vi "Weather Parse Test.vi"() -> ()   [LabVIEW 2020, in "CDM-Config.lvlib"] (continued)
        \"response\": \"Avoid\",\n                \"parameters\": {\n                    \"AWIPSidentifier\": [\n                        \"CWFWCZ\"\n                    ],\n                    \"WMOidentifier\": [\n                        \"FZAK52 PAFG 031247\"\n                    ],\n                    \"NWSheadline\": [\n                        \"GALE WARNING IN EFFECT THROUGH THIS MORNING... ...HEAVY FREEZING SPRAY WARNING IN EFFECT THROUGH LATE TONIGHT\"\n                    ],\n                    \"BLOCKCHANNEL\": [\n                        \"EAS\",\n                        \"NWEM\",\n                        \"CMAS\"\n                    ],\n                    \"VTEC\": [\n                        \"/O.NEW.PAFG.UP.W.8907.251203T1200Z-251204T1400Z/\"\n                    ],\n                    \"eventEndingTime\": [\n                        \"2025-12-04T05:00:00-09:00\"\n                    ]\n                },\n                \"scope\": \"Public\",\n                \"code\": \"IPAWSv1.0\",\n                \"language\": \"en-US\",\n                \"web\": \"http://www.weather.gov\",\n                \"eventCode\": {\n                    \"SAME\": [\n                        \"NWS\"\n                    ],\n                    \"NationalWeatherService\": [\n                        \"UPW\"\n                    ]\n                }\n            }\n        },\n        {\n            \"id\": \"https://api.weather.gov/alerts/urn:oid:2.49.0.1.840.0.c800d83de15e9a71d59e2d9241e36be98ce51c45.005.1\",\n            \"type\": \"Feature\",\n            \"geometry\": null,\n            \"properties\": {\n                \"@id\": \"https://api.weather.gov/alerts/urn:oid:2.49.0.1.840.0.c800d83de15e9a71d59e2d9241e36be98ce51c45.005.1\",\n                \"@type\": \"wx:Alert\",\n                \"id\": \"urn:oid:2.49.0.1.840.0.c800d83de15e9a71d59e2d9241e36be98ce51c45.005.1\",\n                \"areaDesc\": \"Flaxman Island to Demarcation Point out to 15 NM\",\n                \"geocode\": {\n                    \"SAME\": [\n                        \"058815\"\n                    ],\n                    \"UGC\": [\n                        \"PKZ815\"\n                    ]\n                },\n                \"affectedZones\": [\n                    \"https://api.weather.gov/zones/forecast/PKZ815\"\n                ],\n                \"references\": [],\n                \"sent\": \"2025-12-03T03:46:00-09:00\",\n                \"effective\": \"2025-12-03T03:45:00-09:00\",\n                \"onset\": \"2025-12-03T03:00:00-09:00\",\n                \"expires\": \"2025-12-03T18:00:00-09:00\",\n                \"ends\": \"2025-12-04T05:00:00-09:00\",\n                \"status\": \"Actual\",\n                \"messageType\": \"Alert\",\n                \"category\": \"Met\",\n                \"severity\": \"Minor\",\n                \"certainty\": \"Likely\",\n                \"urgency\": \"Expected\",\n                \"event\": \"Brisk Wind Advisory\",\n                \"sender\": \"w-nws.webmaster@noaa.gov\",\n                \"senderName\": \"NWS Fairbanks AK\",\n                \"headline\": \"Brisk Wind Advisory issued December 3 at 3:45AM AKST until December 4 at 5:00AM AKST by NWS Fairbanks AK\",\n                \"description\": \"Arctic Alaska Coastal Waters out 100 NM\\n\\nWind forecasts reflect the predominant speed and direction\\nexpected. Sea forecasts represent the average of the highest one-\\nthird of the combined wind-wave and swell height.\\n\\n.TODAY...W winds 25 kt.\\n.TONIGHT...W winds 25 kt.\\n.THU...W winds 10 kt.\\n.THU NIGHT...W winds 10 kt.\\n.FRI...NW winds 10 kt.\\n.FRI NIGHT...NW winds 10 kt.\\n.SAT...W winds 10 kt.\\n.SUN...W winds 10 kt.\",\n                \"instruction\": null,\n                \"response\": \"Avoid\",\n                \"parameters\": {\n                    \"AWIPSidentifier\": [\n                        \"CWFNSB\"\n                    ],\n                    \"WMOidentifier\": [\n                        \"FZAK51 PAFG 031246\"\n                    ],\n                    \"NWSheadline\": [\n                        \"BRISK WIND ADVISORY IN EFFECT THROUGH LATE TONIGHT\"\n                    ],\n                    \"BLOCKCHANNEL\": [\n                        \"EAS\",\n                        \"NWEM\",\n                        \"CMAS\"\n                    ],\n                    \"VTEC\": [\n                        \"/O.NEW.PAFG.BW.Y.7401.251203T1200Z-251204T1400Z/\"\n                    ],\n                    \"eventEndingTime\": [\n                        \"2025-12-04T05:00:00-09:00\"\n                    ]\n                },\n                \"scope\": \"Public\",\n                \"code\": \"IPAWSv1.0\",\n                \"language\": \"en-US\",\n                \"web\": \"http://www.weather.gov\",\n                \"eventCode\": {\n                    \"SAME\": [\n                        \"NWS\"\n                    ],\n                    \"NationalWeatherService\": [\n                        \"BWY\"\n                    ]\n                }\n            }\n        },\n        {\n            \"id\": \"https://api.weather.gov/alerts/urn:oid:2.49.0.1.840.0.c800d83de15e9a71d59e2d9241e36be98ce51c45.010.1\",\n            \"type\": \"Feature\",\n            \"geometry\": null,\n            \"properties\": {\n                \"@id\": \"https://api.weather.gov/alerts/urn:oid:2.49.0.1.840.0.c800d83de15e9a71d59e2d9241e36be98ce51c45.010.1\",\n                \"@type\": \"wx:Alert\",\n                \"id\": \"urn:oid:2.49.0.1.840.0.c800d83de15e9a71d59e2d9241e36be98ce51c45.010.1\",\n                \"areaDesc\": \"Flaxman Island to Demarcation Point from 15 to 75 NM\",\n                \"geocode\": {\n                    \"SAME\": [\n                        \"058861\"\n                    ],\n                    \"UGC\": [\n                        \"PKZ861\"\n                    ]\n                },\n                \"affectedZones\": [\n                    \"https://api.weather.gov/zones/forecast/PKZ861\"\n                ],\n                \"references\": [],\n                \"sent\": \"2025-12-03T03:46:00-09:00\",\n                \"effective\": \"2025-12-03T03:45:00-09:00\",\n                \"onset\": \"2025-12-03T03:00:00-09:00\",\n                \"expires\": \"2025-12-03T18:00:00-09:00\",\n                \"ends\": \"2025-12-04T05:00:00-09:00\",\n                \"status\": \"Actual\",\n                \"messageType\": \"Alert\",\n                \"category\": \"Met\",\n                \"severity\": \"Minor\",\n                \"certainty\": \"Likely\",\n                \"urgency\": \"Expected\",\n                \"event\": \"Brisk Wind Advisory\",\n                \"sender\": \"w-nws.webmaster@noaa.gov\",\n                \"senderName\": \"NWS Fairbanks AK\",\n                \"headline\": \"Brisk Wind Advisory issued December 3 at 3:45AM AKST until December 4 at 5:00AM AKST by NWS Fairbanks AK\",\n                \"description\": \"Arctic Alaska Coastal Waters out 100 NM\\n\\nWind forecasts reflect the predominant speed and direction\\nexpected. Sea forecasts represent the average of the highest one-\\nthird of the combined wind-wave and swell height.\\n\\n.TODAY...W winds 25 kt.\\n.TONIGHT...W winds 25 kt.\\n.THU...W winds 15 kt.\\n.THU NIGHT...W winds 10 kt.\\n.FRI...NW winds 10 kt.\\n.FRI NIGHT...N winds 10 kt.\\n.SAT...NW winds 10 kt.\\n.SUN...NW winds 10 kt.\",\n                \"instruction\": null,\n                \"response\": \"Avoid\",\n                \"parameters\": {\n                    \"AWIPSidentifier\": [\n                        \"CWFNSB\"\n                    ],\n                    \"WMOidentifier\": [\n                        \"FZAK51 PAFG 031246\"\n                    ],\n                    \"NWSheadline\": [\n                        \"BRISK WIND ADVISORY IN EFFECT THROUGH LATE TONIGHT\"\n                    ],\n                    \"BLOCKCHANNEL\": [\n                        \"EAS\",\n                        \"NWEM\",\n                        \"CMAS\"\n                    ],\n                    \"VTEC\": [\n                        \"/O.NEW.PAFG.BW.Y.7402.251203T1200Z-251204T1400Z/\"\n                    ],\n                    \"eventEndingTime\": [\n                        \"2025-12-04T05:00:00-09:00\"\n                    ]\n                },\n                \"scope\": \"Public\",\n                \"code\": \"IPAWSv1.0\",\n                \"language\": \"en-US\",\n                \"web\": \"http://www.weather.gov\",\n                \"eventCode\": {\n                    \"SAME\": [\n                        \"NWS\"\n                    ],\n                    \"NationalWeatherService\": [\n                        \"BWY\"\n                    ]\n                }\n            }\n        },\n        {\n            \"id\": \"https://api.weather.gov/alerts/urn:oid:2.49.0.1.840.0.01783fcbff0a57acfaa8774dbd3d755b2c9bae1b.005.1\",\n            \"type\": \"Feature\",\n            \"geometry\": null,\n            \"properties\": {\n                \"@id\": \"https://api.weather.gov/alerts/urn:oid:2.49.0.1.840.0.01783fcbff0a57acfaa8774dbd3d755b2c9bae1b.005.1\",\n                \"@type\": \"wx:Alert\",\n                \"id\": \"urn:oid:2.49.0.1.840.0.01783fcbff0a57acfaa8774dbd3d755b2c9bae1b.005.1\",\n                \"areaDesc\": \"Boulder And Jefferson Counties Below 6000 Feet/West Broomfield County; North Douglas County Below 6000 Feet/Denver/West Adams and Arapahoe Counties/East Broomfield County; Elbert/Central and East Douglas Counties Above 6000 Feet\",\n                \"geocode\": {\n                    \"SAME\": [\n                        \"008013\",\n                        \"008014\",\n                        \"008059\",\n                        \"008001\",\n                        \"008005\",\n                        \"008031\",\n                        \"008035\",\n                        \"008039\"\n                    ],\n                    \"UGC\": [\n                        \"COZ039\",\n                        \"COZ040\",\n                        \"COZ041\"\n                    ]\n                },\n                \"affectedZones\": [\n                    \"https://api.weather.gov/zones/forecast/COZ039\",\n                    \"https://api.weather.gov/zones/forecast/COZ040\",\n                    \"https://api.weather.gov/zones/forecast/COZ041\"\n                ],\n                \"references\": [\n                    {\n                        \"@id\": \"https://api.weather.gov/alerts/urn:oid:2.49.0.1.840.0.dc493d5144a5e7b208e25eb0a352a3a4cb8daa39.005.1\",\n                        \"identifier\": \"urn:oid:2.49.0.1.840.0.dc493d5144a5e7b208e25eb0a352a3a4cb8daa39.005.1\",\n                        \"sender\": \"w-nws.webmaster@noaa.gov\",\n                        \"sent\": \"2025-12-02T14:37:00-07:00\"\n                    },\n                    {\n                        \"@id\": \"https://api.weather.gov/alerts/urn:oid:2.49.0.1.840.0.9981ab0aab6442180ca93df6a3f6876711e70914.004.1\",\n                        \"identifier\": \"urn:oid:2.49.0.1.840.0.9981ab0aab6442180ca93df6a3f6876711e70914.004.1\",\n                        \"sender\": \"w-nws.webmaster@noaa.gov\",\n                        \"sent\": \"2025-12-02T22:13:00-07:00\"\n                    }\n                ],\n                \"sent\": \"2025-12-03T05:02:00-07:00\",\n                \"effective\": \"2025-12-03T05:02:00-07:00\",\n                \"onset\": \"2025-12-03T05:02:00-07:00\",\n                \"expires\": \"2025-12-03T13:15:00-07:00\",\n                \"ends\": \"2025-12-03T18:00:00-07:00\",\n                \"status\": \"Actual\",\n                \"messageType\": \"Update\",\n                \"category\": \"Met\",\n                \"severity\": \"Moderate\",\n                \"certainty\": \"Likely\",\n                \"urgency\": \"Expected\",\n                \"event\": \"Winter Weather Advisory\",\n                \"sender\": \"w-nws.webmaster@noaa.gov\",\n                \"senderName\": \"NWS Denver CO\",\n                \"headline\": \"Winter Weather Advisory issued December 3 at 5:02AM MST until December 3 at 6:00PM MST by NWS Denver CO\",\n                \"description\": \"* WHAT...Snow. Additional snow accumulations between 1 and 4 inches,\\nwith storm totals ranging from 3 to 6 inches. The heavier totals\\nwill be west of I-25. Locally heavier amounts close to 8 inches\\nwill be possible at the base of the foothills.\\n\\n* WHERE...Boulder and Denver metro areas, Castle Rock, and Palmer\\nDivide.\\n\\n* WHEN...Until 6 PM MST this evening.\\n\\n* IMPACTS...Plan on slippery road conditions and slow travel. The\\nhazardous conditions will impact the Wednesday morning commute,\\nwith potential for slick roads to persist into the evening commute\\nas well.\",\n                \"instruction\": \"Slow down and use caution while traveling. The latest road conditions\\nfor Colorado can be obtained by calling 5 1 1 or by going to\\nwww.cotrip.org.\",\n                \"response\": \"Execute\",\n                \"parameters\": {\n                    \"AWIPSidentifier\": [\n                        \"WSWBOU\"\n                    ],\n                    \"WMOidentifier\": [\n                        \"WWUS45 KBOU 031202\"\n                    ],\n                    \"NWSheadline\": [\n                        \"WINTER WEATHER ADVISORY REMAINS IN EFFECT UNTIL 6 PM MST THIS EVENING\"\n                    ],\n                    \"BLOCKCHANNEL\": [\n                        \"EAS\",\n                        \"NWEM\",\n                        \"CMAS\"\n                    ],\n                    \"VTEC\": [\n                        \"/O.CON.KBOU.WW.Y.0029.000000T0000Z-251204T0100Z/\"\n                    ],\n                    \"eventEndingTime\": [\n                        \"2025-12-03T18:00:00-07:00\"\n                    ],\n                    \"expiredReferences\": [\n                        \"w-nws.webmaster@noaa.gov,urn:oid:2.49.0.1.840.0.a94969ba77db5be5a7a7221a7b90d8c1f14402d8.002.1,2025-12-02T02:53:00-07:00 w-nws.webmaster@noaa.gov,urn:oid:2.49.0.1.840.0.e69a2f297fcb0f2a4247bcda904ffb3742464c99.001.1,2025-12-01T13:52:00-07:00\"\n                    ]\n                },\n                \"scope\": \"Public\",\n                \"code\": \"IPAWSv1.0\",\n                \"language\": \"en-US\",\n                \"web\": \"http://www.weather.gov\",\n                \"eventCode\": {\n                    \"SAME\": [\n                        \"NWS\"\n                    ],\n                    \"NationalWeatherService\": [\n                        \"WWY\"\n                    ]\n                }\n            }\n        },\n        {\n            \"id\": \"https://api.weather.gov/alerts/urn:oid:2.49.0.1.840.0.01783fcbff0a57acfaa8774dbd3d755b2c9bae1b.003.1\",\n            \"type\": \"Feature\",\n            \"geometry\": null,\n            \"properties\": {\n                \"@id\": \"https://api.weather.gov/alerts/urn:oid:2.49.0.1.840.0.01783fcbff0a57acfaa8774dbd3d755b2c9bae1b.003.1\",\n                \"@type\": \"wx:Alert\",\n                \"id\": \"urn:oid:2.49.0.1.840.0.01783fcbff0a57acfaa8774dbd3d755b2c9bae1b.003.1\",\n                \"areaDesc\": \"Central and Southeast Park County\",\n                \"geocode\": {\n                    \"SAME\": [\n                        \"008093\"\n                    ],\n                    \"UGC\": [\n                        \"COZ037\"\n                    ]\n                },\n                \"affectedZones\": [\n                    \"https://api.weather.gov/zones/forecast/COZ037\"\n                ],\n                \"references\": [\n                    {\n                        \"@id\": \"https://api.weather.gov/alerts/urn:oid:2.49.0.1.840.0.dc493d5144a5e7b208e25eb0a352a3a4cb8daa39.002.1\",\n                        \"identifier\": \"urn:oid:2.49.0.1.840.0.dc493d5144a5e7b208e25eb0a352a3a4cb8daa39.002.1\",\n                        \"sender\": \"w-nws.webmaster@noaa.gov\",\n                        \"sent\": \"2025-12-02T14:37:00-07:00\"\n                    },\n                    {\n                        \"@id\": \"https://api.weather.gov/alerts/urn:oid:2.49.0.1.840.0.9981ab0aab6442180ca93df6a3f6876711e70914.005.1\",\n                        \"identifier\": \"urn:oid:2.49.0.1.840.0.9981ab0aab6442180ca93df6a3f6876711e70914.005.1\",\n                        \"sender\": \"w-nws.webmaster@noaa.gov\",\n                        \"sent\": \"2025-12-02T22:13:00-07:00\"\n                    }\n                ],\n                \"sent\": \"2025-12-03T05:02:00-07:00\",\n                \"effective\": \"2025-12-03T05:02:00-07:00\",\n                \"onset\": \"2025-12-03T05:02:00-07:00\",\n                \"expires\": \"2025-12-03T13:15:00-07:00\",\n                \"ends\": \"2025-12-03T20:00:00-07:00\",\n                \"status\": \"Actual\",\n                \"messageType\": \"Update\",\n                \"category\": \"Met\",\n                \"severity\": \"Moderate\",\n                \"certainty\": \"Likely\",\n                \"urgency\": \"Expected\",\n                \"event\": \"Winter Weather Advisory\",\n                \"sender\": \"w-nws.webmaster@noaa.gov\",\n                \"senderName\": \"NWS Denver CO\",\n                \"headline\": \"Winter Weather Advisory issued December 3 at 5:02AM MST until December 3 at 8:00PM MST by NWS Denver CO\",\n                \"description\": \"* WHAT...Snow expected. Total snow accumulations between 3 and 8\\ninches.\\n\\n* WHERE...South Park.\\n\\n* WHEN...Until 8 PM MST this evening.\\n\\n* IMPACTS...Travel will be hazardous with slippery road conditions.\",\n                \"instruction\": \"Slow down and use caution while traveling. The latest road conditions\\nfor Colorado can be obtained by calling 5 1 1 or by going to\\nwww.cotrip.org.\",\n                \"response\": \"Execute\",\n                \"parameters\": {\n                    \"AWIPSidentifier\": [\n                        \"WSWBOU\"\n                    ],\n                    \"WMOidentifier\": [\n                        \"WWUS45 KBOU 031202\"\n                    ],\n                    \"NWSheadline\": [\n                        \"WINTER WEATHER ADVISORY REMAINS IN EFFECT UNTIL 8 PM MST THIS EVENING\"\n                    ],\n                    \"BLOCKCHANNEL\": [\n                        \"EAS\",\n                        \"NWEM\",\n                        \"CMAS\"\n                    ],\n                    \"VTEC\": [\n                        \"/O.CON.KBOU.WW.Y.0029.000000T0000Z-251204T0300Z/\"\n                    ],\n                    \"eventEndingTime\": [\n                        \"2025-12-03T20:00:00-07:00\"\n                    ]\n                },\n                \"scope\": \"Public\",\n                \"code\": \"IPAWSv1.0\",\n                \"language\": \"en-US\",\n                \"web\": \"http://www.weather.gov\",\n                \"eventCode\": {\n                    \"SAME\": [\n                        \"NWS\"\n                    ],\n                    \"NationalWeatherService\": [\n                        \"WWY\"\n                    ]\n                }\n            }\n        },\n        {\n            \"id\": \"https://api.weather.gov/alerts/urn:oid:2.49.0.1.840.0.01783fcbff0a57acfaa8774dbd3d755b2c9bae1b.002.1\",\n            \"type\": \"Feature\",\n            \"geometry\": null,\n            \"properties\": {\n                \"@id\": \"https://api.weather.gov/alerts/urn:oid:2.49.0.1.840.0.01783fcbff0a57acfaa8774dbd3d755b2c9bae1b.002.1\",\n                \"@type\": \"wx:Alert\",\n                \"id\": \"urn:oid:2.49.0.1.840.0.01783fcbff0a57acfaa8774dbd3d755b2c9bae1b.002.1\",\n                \"areaDesc\": \"Jefferson and West Douglas Counties Above  6000 Feet/Gilpin/Clear Creek/Northeast Park Counties Below 9000 Feet\",\n                \"geocode\": {\n                    \"SAME\": [\n                        \"008019\",\n                        \"008035\",\n                        \"008047\",\n                        \"008059\",\n                        \"008093\"\n                    ],\n                    \"UGC\": [\n                        \"COZ036\"\n                    ]\n                },\n                \"affectedZones\": [\n                    \"https://api.weather.gov/zones/forecast/COZ036\"\n                ],\n                \"references\": [\n                    {\n                        \"@id\": \"https://api.weather.gov/alerts/urn:oid:2.49.0.1.840.0.dc493d5144a5e7b208e25eb0a352a3a4cb8daa39.004.1\",\n                        \"identifier\": \"urn:oid:2.49.0.1.840.0.dc493d5144a5e7b208e25eb0a352a3a4cb8daa39.004.1\",\n                        \"sender\": \"w-nws.webmaster@noaa.gov\",\n                        \"sent\": \"2025-12-02T14:37:00-07:00\"\n                    },\n                    {\n                        \"@id\": \"https://api.weather.gov/alerts/urn:oid:2.49.0.1.840.0.9981ab0aab6442180ca93df6a3f6876711e70914.002.1\",\n                        \"identifier\": \"urn:oid:2.49.0.1.840.0.9981ab0aab6442180ca93df6a3f6876711e70914.002.1\",\n                        \"sender\": \"w-nws.webmaster@noaa.gov\",\n                        \"sent\": \"2025-12-02T22:13:00-07:00\"\n                    }\n                ],\n                \"sent\": \"2025-12-03T05:02:00-07:00\",\n                \"effective\": \"2025-12-03T05:02:00-07:00\",\n                \"onset\": \"2025-12-03T05:02:00-07:00\",\n                \"expires\": \"2025-12-03T13:15:00-07:00\",\n                \"ends\": \"2025-12-03T18:00:00-07:00\",\n                \"status\": \"Actual\",\n                \"messageType\": \"Update\",\n                \"category\": \"Met\",\n                \"severity\": \"Moderate\",\n                \"certainty\": \"Likely\",\n                \"urgency\": \"Expected\",\n                \"event\": \"Winter Weather Advisory\",\n                \"sender\": \"w-nws.webmaster@noaa.gov\",\n                \"senderName\": \"NWS Denver CO\",\n                \"headline\": \"Winter Weather Advisory issued December 3 at 5:02AM MST until December 3 at 6:00PM MST by NWS Denver CO\",\n                \"description\": \"* WHAT...Snow. Additional snow accumulations between 3 and 8 inches,\\nbringing storm totals into the 6 to 11 inch range.\\n\\n* WHERE...The Southern Front Range Foothills.\\n\\n* WHEN...Until 6 PM MST this evening.\\n\\n* IMPACTS...Travel could be difficult. The hazardous conditions will\\nimpact the Wednesday morning and afternoon commutes.\",\n                \"instruction\": \"Slow down and use caution while traveling. The latest road conditions\\nfor Colorado can be obtained by calling 5 1 1 or by going to\\nwww.cotrip.org.\",\n                \"response\": \"Execute\",\n                \"parameters\": {\n                    \"AWIPSidentifier\": [\n                        \"WSWBOU\"\n                    ],\n                    \"WMOidentifier\": [\n                        \"WWUS45 KBOU 031202\"\n                    ],\n                    \"NWSheadline\": [\n                        \"WINTER WEATHER ADVISORY REMAINS IN EFFECT UNTIL 6 PM MST THIS EVENING\"\n                    ],\n                    \"BLOCKCHANNEL\": [\n                        \"EAS\",\n                        \"NWEM\",\n                        \"CMAS\"\n                    ],\n                    \"VTEC\": [\n                        \"/O.CON.KBOU.WW.Y.0029.000000T0000Z-251204T0100Z/\"\n                    ],\n                    \"eventEndingTime\": [\n                        \"2025-12-03T18:00:00-07:00\"\n                    ],\n                    \"expiredReferences\": [\n                        \"w-nws.webmaster@noaa.gov,urn:oid:2.49.0.1.840.0.a94969ba77db5be5a7a7221a7b90d8c1f14402d8.001.1,2025-12-02T02:53:00-07:00 w-nws.webmaster@noaa.gov,urn:oid:2.49.0.1.840.0.e69a2f297fcb0f2a4247bcda904ffb3742464c99.001.1,2025-12-01T13:52:00-07:00\"\n                    ]\n                },\n                \"scope\": \"Public\",\n                \"code\": \"IPAWSv1.0\",\n                \"language\": \"en-US\",\n                \"web\": \"http://www.weather.gov\",\n                \"eventCode\": {\n                    \"SAME\": [\n                        \"NWS\"\n                    ],\n                    \"NationalWeatherService\": [\n                        \"WWY\"\n                    ]\n                }\n            }\n        },\n        {\n            \"id\": \"https://api.weather.gov/alerts/urn:oid:2.49.0.1.840.0.01783fcbff0a57acfaa8774dbd3d755b2c9bae1b.001.1\",\n            \"type\": \"Feature\",\n            \"geometry\": null,\n            \"properties\": {\n                \"@id\": \"https://api.weather.gov/alerts/urn:oid:2.49.0.1.840.0.01783fcbff0a57acfaa8774dbd3d755b2c9bae1b.001.1\",\n                \"@type\": \"wx:Alert\",\n                \"id\": \"urn:oid:2.49.0.1.840.0.01783fcbff0a57acfaa8774dbd3d755b2c9bae1b.001.1\",\n                \"areaDesc\": \"Larimer and Boulder Counties Between 6000 and 9000 Feet\",\n                \"geocode\": {\n                    \"SAME\": [\n                        \"008013\",\n                        \"008069\"\n                    ],\n                    \"UGC\": [\n                        \"COZ035\"\n                    ]\n                },\n                \"affectedZones\": [\n                    \"https://api.weather.gov/zones/forecast/COZ035\"\n                ],\n                \"references\": [\n                    {\n                        \"@id\": \"https://api.weather.gov/alerts/urn:oid:2.49.0.1.840.0.dc493d5144a5e7b208e25eb0a352a3a4cb8daa39.003.1\",\n                        \"identifier\": \"urn:oid:2.49.0.1.840.0.dc493d5144a5e7b208e25eb0a352a3a4cb8daa39.003.1\",\n                        \"sender\": \"w-nws.webmaster@noaa.gov\",\n                        \"sent\": \"2025-12-02T14:37:00-07:00\"\n                    },\n                    {\n                        \"@id\": \"https://api.weather.gov/alerts/urn:oid:2.49.0.1.840.0.9981ab0aab6442180ca93df6a3f6876711e70914.001.1\",\n                        \"identifier\": \"urn:oid:2.49.0.1.840.0.9981ab0aab6442180ca93df6a3f6876711e70914.001.1\",\n                        \"sender\": \"w-nws.webmaster@noaa.gov\",\n                        \"sent\": \"2025-12-02T22:13:00-07:00\"\n                    }\n                ],\n                \"sent\": \"2025-12-03T05:02:00-07:00\",\n                \"effective\": \"2025-12-03T05:02:00-07:00\",\n                \"onset\": \"2025-12-03T05:02:00-07:00\",\n                \"expires\": \"2025-12-03T13:15:00-07:00\",\n                \"ends\": \"2025-12-03T18:00:00-07:00\",\n                \"status\": \"Actual\",\n                \"messageType\": \"Update\",\n                \"category\": \"Met\",\n                \"severity\": \"Moderate\",\n                \"certainty\": \"Likely\",\n                \"urgency\": \"Expected\",\n                \"event\": \"Winter Weather Advisory\",\n                \"sender\": \"w-nws.webmaster@noaa.gov\",\n                \"senderName\": \"NWS Denver CO\",\n                \"headline\": \"Winter Weather Advisory issued December 3 at 5:02AM MST until December 3 at 6:00PM MST by NWS Denver CO\",\n                \"description\": \"* WHAT...Snow. Additional snow accumulations between 2 and 4 inches,\\nbringing storm totals to between 3 and 9 inches. The heaviest\\namounts will be in the Boulder County Foothills, with lighter\\namounts in northern Larimer County.\\n\\n* WHERE...The Northern Front Range Foothills.\\n\\n* WHEN...Until 6 PM MST this evening.\\n\\n* IMPACTS...Travel could be difficult. The hazardous conditions will\\nimpact the Wednesday morning commute.\",\n                \"instruction\": \"Slow down and use caution while traveling. The latest road conditions\\nfor Colorado can be obtained by calling 5 1 1 or by going to\\nwww.cotrip.org.\",\n                \"response\": \"Execute\",\n                \"parameters\": {\n                    \"AWIPSidentifier\": [\n                        \"WSWBOU\"\n                    ],\n                    \"WMOidentifier\": [\n                        \"WWUS45 KBOU 031202\"\n                    ],\n                    \"NWSheadline\": [\n                        \"WINTER WEATHER ADVISORY REMAINS IN EFFECT UNTIL 6 PM MST THIS EVENING\"\n                    ],\n                    \"BLOCKCHANNEL\": [\n                        \"EAS\",\n                        \"NWEM\",\n                        \"CMAS\"\n                    ],\n                    \"VTEC\": [\n                        \"/O.CON.KBOU.WW.Y.0029.000000T0000Z-251204T0100Z/\"\n                    ],\n                    \"eventEndingTime\": [\n                        \"2025-12-03T18:00:00-07:00\"\n                    ]\n                },\n                \"scope\": \"Public\",\n                \"code\": \"IPAWSv1.0\",\n                \"language\": \"en-US\",\n                \"web\": \"http://www.weather.gov\",\n                \"eventCode\": {\n                    \"SAME\": [\n                        \"NWS\"\n                    ],\n                    \"NationalWeatherService\": [\n                        \"WWY\"\n                    ]\n                }\n            }\n        },\n        {\n            \"id\": \"https://api.weather.gov/alerts/urn:oid:2.49.0.1.840.0.01783fcbff0a57acfaa8774dbd3d755b2c9bae1b.004.1\",\n            \"type\": \"Feature\",\n            \"geometry\": null,\n            \"properties\": {\n                \"@id\": \"https://api.weather.gov/alerts/urn:oid:2.49.0.1.840.0.01783fcbff0a57acfaa8774dbd3d755b2c9bae1b.004.1\",\n                \"@type\": \"wx:Alert\",\n                \"id\": \"urn:oid:2.49.0.1.840.0.01783fcbff0a57acfaa8774dbd3d755b2c9bae1b.004.1\",\n                \"areaDesc\": \"Larimer County Below 6000 Feet/Northwest Weld County\",\n                \"geocode\": {\n                    \"SAME\": [\n                        \"008069\",\n                        \"008123\"\n                    ],\n                    \"UGC\": [\n                        \"COZ038\"\n                    ]\n                },\n                \"affectedZones\": [\n                    \"https://api.weather.gov/zones/forecast/COZ038\"\n                ],\n                \"references\": [\n                    {\n                        \"@id\": \"https://api.weather.gov/alerts/urn:oid:2.49.0.1.840.0.dc493d5144a5e7b208e25eb0a352a3a4cb8daa39.001.1\",\n                        \"identifier\": \"urn:oid:2.49.0.1.840.0.dc493d5144a5e7b208e25eb0a352a3a4cb8daa39.001.1\",\n                        \"sender\": \"w-nws.webmaster@noaa.gov\",\n                        \"sent\": \"2025-12-02T14:37:00-07:00\"\n                    },\n                    {\n                        \"@id\": \"https://api.weather.gov/alerts/urn:oid:2.49.0.1.840.0.9981ab0aab6442180ca93df6a3f6876711e70914.003.1\",\n                        \"identifier\": \"urn:oid:2.49.0.1.840.0.9981ab0aab6442180ca93df6a3f6876711e70914.003.1\",\n                        \"sender\": \"w-nws.webmaster@noaa.gov\",\n                        \"sent\": \"2025-12-02T22:13:00-07:00\"\n                    }\n                ],\n                \"sent\": \"2025-12-03T05:02:00-07:00\",\n                \"effective\": \"2025-12-03T05:02:00-07:00\",\n                \"onset\": \"2025-12-03T05:02:00-07:00\",\n                \"expires\": \"2025-12-03T13:15:00-07:00\",\n                \"ends\": \"2025-12-03T14:00:00-07:00\",\n                \"status\": \"Actual\",\n                \"messageType\": \"Update\",\n                \"category\": \"Met\",\n                \"severity\": \"Moderate\",\n                \"certainty\": \"Likely\",\n                \"urgency\": \"Expected\",\n                \"event\": \"Winter Weather Advisory\",\n                \"sender\": \"w-nws.webmaster@noaa.gov\",\n                \"senderName\": \"NWS Denver CO\",\n                \"headline\": \"Winter Weather Advisory issued December 3 at 5:02AM MST until December 3 at 2:00PM MST by NWS Denver CO\",\n                \"description\": \"* WHAT...Snow. Additional snow accumulations less than two inches,\\nwith storm totals mostly between 2 and 5 inches.\\n\\n* WHERE...Fort Collins and Loveland.\\n\\n* WHEN...Until 2 PM MST this afternoon.\\n\\n* IMPACTS...Plan on slippery road conditions and slow travel. The\\nhazardous conditions will impact the Wednesday morning commute,\\nwith potential for slick roads to persist into the evening commute\\nas well.\",\n                \"instruction\": \"Slow down and use caution while traveling. The latest road conditions\\nfor Colorado can be obtained by calling 5 1 1 or by going to\\nwww.cotrip.org.\",\n                \"response\": \"Execute\",\n                \"parameters\": {\n                    \"AWIPSidentifier\": [\n                        \"WSWBOU\"\n                    ],\n                    \"WMOidentifier\": [\n                        \"WWUS45 KBOU 031202\"\n                    ],\n                    \"NWSheadline\": [\n                        \"WINTER WEATHER ADVISORY REMAINS IN EFFECT UNTIL 2 PM MST THIS AFTERNOON\"\n                    ],\n                    \"BLOCKCHANNEL\": [\n                        \"EAS\",\n                        \"NWEM\",\n                        \"CMAS\"\n                    ],\n                    \"VTEC\": [\n                        \"/O.CON.KBOU.WW.Y.0029.000000T0000Z-251203T2100Z/\"\n                    ],\n                    \"eventEndingTime\": [\n                        \"2025-12-03T14:00:00-07:00\"\n                    ]\n                },\n                \"scope\": \"Public\",\n                \"code\": \"IPAWSv1.0\",\n                \"language\": \"en-US\",\n                \"web\": \"http://www.weather.gov\",\n                \"eventCode\": {\n                    \"SAME\": [\n                        \"NWS\"\n                    ],\n                    \"NationalWeatherService\": [\n                        \"WWY\"\n                    ]\n                }\n            }\n        },\n        {\n            \"id\": \"https://api.weather.gov/alerts/urn:oid:2.49.0.1.840.0.98086d1e66fc68dd47444e78c2dfcce526122be3.002.1\",\n            \"type\": \"Feature\",\n            \"geometry\": null,\n            \"properties\": {\n                \"@id\": \"https://api.weather.gov/alerts/urn:oid:2.49.0.1.840.0.98086d1e66fc68dd47444e78c2dfcce526122be3.002.1\",\n                \"@type\": \"wx:Alert\",\n                \"id\": \"urn:oid:2.49.0.1.840.0.98086d1e66fc68dd47444e78c2dfcce526122be3.002.1\",\n                \"areaDesc\": \"North Bay Interior Valleys; San Francisco Bay Shoreline\",\n                \"geocode\": {\n                    \"SAME\": [\n                        \"006041\",\n                        \"006055\",\n                        \"006097\",\n                        \"006001\",\n                        \"006013\",\n                        \"006081\",\n                        \"006085\"\n                    ],\n                    \"UGC\": [\n                        \"CAZ506\",\n                        \"CAZ508\"\n                    ]\n                },\n                \"affectedZones\": [\n                    \"https://api.weather.gov/zones/forecast/CAZ506\",\n                    \"https://api.weather.gov/zones/forecast/CAZ508\"\n                ],\n                \"references\": [\n                    {\n                        \"@id\": \"https://api.weather.gov/alerts/urn:oid:2.49.0.1.840.0.781259559f375ea2ce2539f3b1491c2c65217487.002.1\",\n                        \"identifier\": \"urn:oid:2.49.0.1.840.0.781259559f375ea2ce2539f3b1491c2c65217487.002.1\",\n                        \"sender\": \"w-nws.webmaster@noaa.gov\",\n                        \"sent\": \"2025-12-02T20:38:00-08:00\"\n                    }\n                ],\n                \"sent\": \"2025-12-03T03:53:00-08:00\",\n                \"effective\": \"2025-12-03T03:53:00-08:00\",\n                \"onset\": \"2025-12-03T03:53:00-08:00\",\n                \"expires\": \"2025-12-03T22:00:00-08:00\",\n                \"ends\": \"2025-12-07T15:00:00-08:00\",\n                \"status\": \"Actual\",\n                \"messageType\": \"Update\",\n                \"category\": \"Met\",\n                \"severity\": \"Minor\",\n                \"certainty\": \"Likely\",\n                \"urgency\": \"Expected\",\n                \"event\": \"Coastal Flood Advisory\",\n                \"sender\": \"w-nws.webmaster@noaa.gov\",\n                \"senderName\": \"NWS San Francisco CA\",\n                \"headline\": \"Coastal Flood Advisory issued December 3 at 3:53AM PST until December 7 at 3:00PM PST by NWS San Francisco CA\",\n                \"description\": \"* WHAT...Up to 1.4 ft of inundation above ground level is\\npossible in low lying areas near shorelines and tidal\\nwaterways.\\n\\n* WHERE...Bayshore locations along the San Francisco Bay and San\\nPablo Bay.\\n\\n* WHEN...Until 3 PM PST Sunday.\\n\\n* IMPACTS...Flooding of lots, parks, and roads with only\\nisolated road closures expected.\\n\\n* ADDITIONAL DETAILS...At the San Francisco tidal gauge high\\ntide is expected to be 1.2 ft above normal (7.00 ft MLLW) at\\n9:04 AM Wednesday, 1.4 ft above normal (7.20 ft MLLW) at 9:48\\nAM Thursday, 1.4 ft above normal (7.23 ft MLLW) at 10:35 AM\\nFriday, 1.2 ft above normal (7.08 ft MLLW) at 11:25 AM\\nSaturday, and 0.9 ft above normal (6.75 ft MLLW) at 12:17 PM\\nSunday. High tide timing varies up to 90 minutes earlier or\\nlater along the Pacific Coast and throughout the San Francisco\\nBay respectively.\",\n                \"instruction\": \"If travel is required, allow extra time as some roads may be\\nclosed. Do not drive around barricades or through water of\\nunknown depth. Take the necessary actions to protect flood-prone\\nproperty.\",\n                \"response\": \"Monitor\",\n                \"parameters\": {\n                    \"AWIPSidentifier\": [\n                        \"CFWMTR\"\n                    ],\n                    \"WMOidentifier\": [\n                        \"WHUS46 KMTR 031153\"\n                    ],\n                    \"NWSheadline\": [\n                        \"COASTAL FLOOD ADVISORY REMAINS IN EFFECT UNTIL 3 PM PST SUNDAY\"\n                    ],\n                    \"BLOCKCHANNEL\": [\n                        \"EAS\",\n                        \"NWEM\",\n                        \"CMAS\"\n                    ],\n                    \"VTEC\": [\n                        \"/O.CON.KMTR.CF.Y.0016.000000T0000Z-251207T2300Z/\"\n                    ],\n                    \"eventEndingTime\": [\n                        \"2025-12-07T15:00:00-08:00\"\n                    ],\n                    \"expiredReferences\": [\n                        \"w-nws.webmaster@noaa.gov,urn:oid:2.49.0.1.840.0.08848c991336157878d38d1ffbfc9e9742984e52.002.1,2025-12-02T08:58:00-08:00 w-nws.webmaster@noaa.gov,urn:oid:2.49.0.1.840.0.af0dcb2190bc14836408315e4cc580c3d2cdeb53.002.1,2025-12-01T18:47:00-08:00 w-nws.webmaster@noaa.gov,urn:oid:2.49.0.1.840.0.21b1376d647bf4746e0a218223471eee19671728.002.1,2025-11-30T22:05:00-08:00 w-nws.webmaster@noaa.gov,urn:oid:2.49.0.1.840.0.1f8316f92149688b39489970d53bd68f7773609a.002.1,2025-11-30T18:54:00-08:00\"\n                    ]\n                },\n                \"scope\": \"Public\",\n                \"code\": \"IPAWSv1.0\",\n                \"language\": \"en-US\",\n                \"web\": \"http://www.weather.gov\",\n                \"eventCode\": {\n                    \"SAME\": [\n                        \"NWS\"\n                    ],\n                    \"NationalWeatherService\": [\n                        \"CFY\"\n                    ]\n                }\n            }\n        },\n        {\n            \"id\": \"https://api.weather.gov/alerts/urn:oid:2.49.0.1.840.0.98086d1e66fc68dd47444e78c2dfcce526122be3.003.1\",\n            \"type\": \"Feature\",\n            \"geometry\": null,\n            \"properties\": {\n                \"@id\": \"https://api.weather.gov/alerts/urn:oid:2.49.0.1.840.0.98086d1e66fc68dd47444e78c2dfcce526122be3.003.1\",\n                \"@type\": \"wx:Alert\",\n                \"id\": \"urn:oid:2.49.0.1.840.0.98086d1e66fc68dd47444e78c2dfcce526122be3.003.1\",\n                \"areaDesc\": \"Coastal North Bay Including Point Reyes National Seashore; San Francisco Peninsula Coast\",\n                \"geocode\": {\n                    \"SAME\": [\n                        \"006041\",\n                        \"006097\",\n                        \"006081\",\n                        \"006087\"\n                    ],\n                    \"UGC\": [\n                        \"CAZ505\",\n                        \"CAZ509\"\n                    ]\n                },\n                \"affectedZones\": [\n                    \"https://api.weather.gov/zones/forecast/CAZ505\",\n                    \"https://api.weather.gov/zones/forecast/CAZ509\"\n                ],\n                \"references\": [\n                    {\n                        \"@id\": \"https://api.weather.gov/alerts/urn:oid:2.49.0.1.840.0.781259559f375ea2ce2539f3b1491c2c65217487.003.1\",\n                        \"identifier\": \"urn:oid:2.49.0.1.840.0.781259559f375ea2ce2539f3b1491c2c65217487.003.1\",\n                        \"sender\": \"w-nws.webmaster@noaa.gov\",\n                        \"sent\": \"2025-12-02T20:38:00-08:00\"\n                    }\n                ],\n                \"sent\": \"2025-12-03T03:53:00-08:00\",\n                \"effective\": \"2025-12-03T03:53:00-08:00\",\n                \"onset\": \"2025-12-03T03:53:00-08:00\",\n                \"expires\": \"2025-12-03T22:00:00-08:00\",\n                \"ends\": \"2025-12-03T22:00:00-08:00\",\n                \"status\": \"Actual\",\n                \"messageType\": \"Update\",\n                \"category\": \"Met\",\n                \"severity\": \"Moderate\",\n                \"certainty\": \"Likely\",\n                \"urgency\": \"Expected\",\n                \"event\": \"Beach Hazards Statement\",\n                \"sender\": \"w-nws.webmaster@noaa.gov\",\n                \"senderName\": \"NWS San Francisco CA\",\n                \"headline\": \"Beach Hazards Statement issued December 3 at 3:53AM PST until December 3 at 10:00PM PST by NWS San Francisco CA\",\n                \"description\": \"* WHAT...Long period westerly swell will result in an increased\\nrisk for sneaker waves and strong rip currents. Breaking waves\\n10 to 14 feet, with long lulls of 10 to 20 minutes or more\\nbetween largest sets.\\n\\n* WHERE...Pacific Coast beaches.\\n\\n* WHEN...Through this evening.\\n\\n* IMPACTS...Sneaker waves can unexpectedly run significantly\\nfarther up the beach than normal, including over rocks and\\njetties. Rip currents are typically more frequent and stronger\\nin the vicinity of jetties, inlets, and piers.\",\n                \"instruction\": \"Dangerous conditions are forecast along the shoreline. Hazards\\ninclude sneaker waves, strong rip currents, and large breaking\\nwaves. Stay off the rocks and NEVER turn your back on the ocean!\",\n                \"response\": \"Avoid\",\n                \"parameters\": {\n                    \"AWIPSidentifier\": [\n                        \"CFWMTR\"\n                    ],\n                    \"WMOidentifier\": [\n                        \"WHUS46 KMTR 031153\"\n                    ],\n                    \"NWSheadline\": [\n                        \"BEACH HAZARDS STATEMENT REMAINS IN EFFECT THROUGH THIS EVENING\"\n                    ],\n                    \"BLOCKCHANNEL\": [\n                        \"EAS\",\n                        \"NWEM\",\n                        \"CMAS\"\n                    ],\n                    \"VTEC\": [\n                        \"/O.CON.KMTR.BH.S.0021.000000T0000Z-251204T0600Z/\"\n                    ],\n                    \"eventEndingTime\": [\n                        \"2025-12-03T22:00:00-08:00\"\n                    ],\n                    \"expiredReferences\": [\n                        \"w-nws.webmaster@noaa.gov,urn:oid:2.49.0.1.840.0.08848c991336157878d38d1ffbfc9e9742984e52.003.1,2025-12-02T08:58:00-08:00 w-nws.webmaster@noaa.gov,urn:oid:2.49.0.1.840.0.af0dcb2190bc14836408315e4cc580c3d2cdeb53.003.1,2025-12-01T18:47:00-08:00 w-nws.webmaster@noaa.gov,urn:oid:2.49.0.1.840.0.21b1376d647bf4746e0a218223471eee19671728.003.1,2025-11-30T22:05:00-08:00 w-nws.webmaster@noaa.gov,urn:oid:2.49.0.1.840.0.1f8316f92149688b39489970d53bd68f7773609a.003.1,2025-11-30T18:54:00-08:00 w-nws.webmaster@noaa.gov,urn:oid:2.49.0.1.840.0.3f4b8992562fc7022a337464b529fc708f287fc3.001.1,2025-11-30T12:17:00-08:00 w-nws.webmaster@noaa.gov,urn:oid:2.49.0.1.840.0.ecd266091eb018733cf4fc9357c5c7fdae77a9b8.001.1,2025-11-30T01:28:00-08:00 w-nws.webmaster@noaa.gov,urn:oid:2.49.0.1.840.0.d12480d3eb90f5fecba0978dd9c1868b1693a420.001.1,2025-11-29T20:46:00-08:00 w-nws.webmaster@noaa.gov,urn:oid:2.49.0.1.840.0.a53d4d7f69e88a6370a59e3493ef574447077913.001.1,2025-11-29T07:30:00-08:00 w-nws.webmaster@noaa.gov,urn:oid:2.49.0.1.840.0.358cf61ddbf1745e21a67e3bba15ca0e524c2b41.001.1,2025-11-28T18:32:00-08:00 w-nws.webmaster@noaa.gov,urn:oid:2.49.0.1.840.0.7e8f6f91e5213f433eda0bb03a347f0857da0a39.001.1,2025-11-28T03:24:00-08:00\"\n                    ]\n                },\n                \"scope\": \"Public\",\n                \"code\": \"IPAWSv1.0\",\n                \"language\": \"en-US\",\n                \"web\": \"http://www.weather.gov\",\n                \"eventCode\": {\n                    \"SAME\": [\n                        \"NWS\"\n                    ],\n                    \"NationalWeatherService\": [\n                        \"BHS\"\n                    ]\n                }\n            }\n        },\n        {\n            \"id\": \"https://api.weather.gov/alerts/urn:oid:2.49.0.1.840.0.98086d1e66fc68dd47444e78c2dfcce526122be3.001.1\",\n            \"type\": \"Feature\",\n            \"geometry\": null,\n            \"properties\": {\n                \"@id\": \"https://api.weather.gov/alerts/urn:oid:2.49.0.1.840.0.98086d1e66fc68dd47444e78c2dfcce526122be3.001.1\",\n                \"@type\": \"wx:Alert\",\n                \"id\": \"urn:oid:2.49.0.1.840.0.98086d1e66fc68dd47444e78c2dfcce526122be3.001.1\",\n                \"areaDesc\": \"San Francisco; Northern Monterey Bay; Southern Monterey Bay and Big Sur Coast\",\n                \"geocode\": {\n                    \"SAME\": [\n                        \"006075\",\n                        \"006087\",\n                        \"006053\"\n                    ],\n                    \"UGC\": [\n                        \"CAZ006\",\n                        \"CAZ529\",\n                        \"CAZ530\"\n                    ]\n                },\n                \"affectedZones\": [\n                    \"https://api.weather.gov/zones/forecast/CAZ006\",\n                    \"https://api.weather.gov/zones/forecast/CAZ529\",\n                    \"https://api.weather.gov/zones/forecast/CAZ530\"\n                ],\n                \"references\": [\n                    {\n                        \"@id\": \"https://api.weather.gov/alerts/urn:oid:2.49.0.1.840.0.781259559f375ea2ce2539f3b1491c2c65217487.001.1\",\n                        \"identifier\": \"urn:oid:2.49.0.1.840.0.781259559f375ea2ce2539f3b1491c2c65217487.001.1\",\n                        \"sender\": \"w-nws.webmaster@noaa.gov\",\n                        \"sent\": \"2025-12-02T20:38:00-08:00\"\n                    }\n                ],\n                \"sent\": \"2025-12-03T03:53:00-08:00\",\n                \"effective\": \"2025-12-03T03:53:00-08:00\",\n                \"onset\": \"2025-12-03T03:53:00-08:00\",\n                \"expires\": \"2025-12-03T22:00:00-08:00\",\n                \"ends\": \"2025-12-07T15:00:00-08:00\",\n                \"status\": \"Actual\",\n                \"messageType\": \"Update\",\n                \"category\": \"Met\",\n                \"severity\": \"Minor\",\n                \"certainty\": \"Likely\",\n                \"urgency\": \"Expected\",\n                \"event\": \"Coastal Flood Advisory\",\n                \"sender\": \"w-nws.webmaster@noaa.gov\",\n                \"senderName\": \"NWS San Francisco CA\",\n                \"headline\": \"Coastal Flood Advisory issued December 3 at 3:53AM PST until December 7 at 3:00PM PST by NWS San Francisco CA\",\n                \"description\": \"* WHAT...For the Beach Hazards Statement, long period westerly\\nswell will result in an increased risk for sneaker waves and\\nstrong rip currents. Breaking waves 10 to 14 feet, with long\\nlulls of 10 to 20 minutes or more between largest sets. For\\nthe Coastal Flood Advisory, up to 1.4 ft of inundation above\\nground level is possible in low lying areas near shorelines\\nand tidal waterways.\\n\\n* WHERE...Bayshore locations along San Francisco and Monterey\\nBay.\\n\\n* WHEN...For the Coastal Flood Advisory, until 3 PM PST Sunday.\\nFor the Beach Hazards Statement, through this evening.\\n\\n* IMPACTS...For the Beach Hazards Statement, sneaker waves can\\nunexpectedly run significantly farther up the beach than\\nnormal, including over rocks and jetties. Rip currents are\\ntypically more frequent and stronger in the vicinity of\\njetties, inlets, and piers. For the Coastal Flood Advisory,\\nflooding of lots, parks, and roads with only isolated road\\nclosures expected.\\n\\n* ADDITIONAL DETAILS...For the Coastal Flood Advisory, at the\\nSan Francisco tidal gauge high tide is expected to be 1.2 ft\\nabove normal (7.00 ft MLLW) at 9:04 AM Wednesday, 1.4 ft above\\nnormal (7.20 ft MLLW) at 9:48 AM Thursday, 1.4 ft above normal\\n(7.23 ft MLLW) at 10:35 AM Friday, 1.2 ft above normal (7.08\\nft MLLW) at 11:25 AM Saturday, and 0.9 ft above normal (6.75\\nft MLLW) at 12:17 PM Sunday. High tide timing varies up to 90\\nminutes earlier or later along the Pacific Coast and\\nthroughout the San Francisco Bay respectively.\",\n                \"instruction\": \"If travel is required, allow extra time as some roads may be\\nclosed. Do not drive around barricades or through water of\\nunknown depth. Take the necessary actions to protect flood-prone\\nproperty.\\n\\nDangerous conditions are forecast along the shoreline. Hazards\\ninclude sneaker waves, strong rip currents, and large breaking\\nwaves. Stay off the rocks and NEVER turn your back on the ocean!\",\n                \"response\": \"Monitor\",\n                \"parameters\": {\n                    \"AWIPSidentifier\": [\n                        \"CFWMTR\"\n                    ],\n                    \"WMOidentifier\": [\n                        \"WHUS46 KMTR 031153\"\n                    ],\n                    \"NWSheadline\": [\n                        \"COASTAL FLOOD ADVISORY REMAINS IN EFFECT UNTIL 3 PM PST SUNDAY... ...BEACH HAZARDS STATEMENT REMAINS IN EFFECT THROUGH THIS EVENING\"\n                    ],\n                    \"BLOCKCHANNEL\": [\n                        \"EAS\",\n                        \"NWEM\",\n                        \"CMAS\"\n                    ],\n                    \"VTEC\": [\n                        \"/O.CON.KMTR.CF.Y.0016.000000T0000Z-251207T2300Z/\"\n                    ],\n                    \"eventEndingTime\": [\n                        \"2025-12-07T15:00:00-08:00\"\n                    ],\n                    \"expiredReferences\": [\n                        \"w-nws.webmaster@noaa.gov,urn:oid:2.49.0.1.840.0.08848c991336157878d38d1ffbfc9e9742984e52.001.1,2025-12-02T08:58:00-08:00 w-nws.webmaster@noaa.gov,urn:oid:2.49.0.1.840.0.af0dcb2190bc14836408315e4cc580c3d2cdeb53.001.1,2025-12-01T18:47:00-08:00 w-nws.webmaster@noaa.gov,urn:oid:2.49.0.1.840.0.21b1376d647bf4746e0a218223471eee19671728.001.2,2025-11-30T22:05:00-08:00 w-nws.webmaster@noaa.gov,urn:oid:2.49.0.1.840.0.1f8316f92149688b39489970d53bd68f7773609a.001.1,2025-11-30T18:54:00-08:00\"\n                    ]\n                },\n                \"scope\": \"Public\",\n                \"code\": \"IPAWSv1.0\",\n                \"language\": \"en-US\",\n                \"web\": \"http://www.weather.gov\",\n                \"eventCode\": {\n                    \"SAME\": [\n                        \"NWS\"\n                    ],\n                    \"NationalWeatherService\": [\n                        \"CFY\"\n                    ]\n                }\n            }\n        },\n        {\n            \"id\": \"https://api.weather.gov/alerts/urn:oid:2.49.0.1.840.0.98086d1e66fc68dd47444e78c2dfcce526122be3.001.2\",\n            \"type\": \"Feature\",\n            \"geometry\": null,\n            \"properties\": {\n                \"@id\": \"https://api.weather.gov/alerts/urn:oid:2.49.0.1.840.0.98086d1e66fc68dd47444e78c2dfcce526122be3.001.2\",\n                \"@type\": \"wx:Alert\",\n                \"id\": \"urn:oid:2.49.0.1.840.0.98086d1e66fc68dd47444e78c2dfcce526122be3.001.2\",\n                \"areaDesc\": \"San Francisco; Northern Monterey Bay; Southern Monterey Bay and Big Sur Coast\",\n                \"geocode\": {\n                    \"SAME\": [\n                        \"006075\",\n                        \"006087\",\n                        \"006053\"\n                    ],\n                    \"UGC\": [\n                        \"CAZ006\",\n                        \"CAZ529\",\n                        \"CAZ530\"\n                    ]\n                },\n                \"affectedZones\": [\n                    \"https://api.weather.gov/zones/forecast/CAZ006\",\n                    \"https://api.weather.gov/zones/forecast/CAZ529\",\n                    \"https://api.weather.gov/zones/forecast/CAZ530\"\n                ],\n                \"references\": [\n                    {\n                        \"@id\": \"https://api.weather.gov/alerts/urn:oid:2.49.0.1.840.0.781259559f375ea2ce2539f3b1491c2c65217487.001.2\",\n                        \"identifier\": \"urn:oid:2.49.0.1.840.0.781259559f375ea2ce2539f3b1491c2c65217487.001.2\",\n                        \"sender\": \"w-nws.webmaster@noaa.gov\",\n                        \"sent\": \"2025-12-02T20:38:00-08:00\"\n                    }\n                ],\n                \"sent\": \"2025-12-03T03:53:00-08:00\",\n                \"effective\": \"2025-12-03T03:53:00-08:00\",\n                \"onset\": \"2025-12-03T03:53:00-08:00\",\n                \"expires\": \"2025-12-03T22:00:00-08:00\",\n                \"ends\": \"2025-12-03T22:00:00-08:00\",\n                \"status\": \"Actual\",\n                \"messageType\": \"Update\",\n                \"category\": \"Met\",\n                \"severity\": \"Moderate\",\n                \"certainty\": \"Likely\",\n                \"urgency\": \"Expected\",\n                \"event\": \"Beach Hazards Statement\",\n                \"sender\": \"w-nws.webmaster@noaa.gov\",\n                \"senderName\": \"NWS San Francisco CA\",\n                \"headline\": \"Beach Hazards Statement issued December 3 at 3:53AM PST until December 3 at 10:00PM PST by NWS San Francisco CA\",\n                \"description\": \"* WHAT...For the Beach Hazards Statement, long period westerly\\nswell will result in an increased risk for sneaker waves and\\nstrong rip currents. Breaking waves 10 to 14 feet, with long\\nlulls of 10 to 20 minutes or more between largest sets. For\\nthe Coastal Flood Advisory, up to 1.4 ft of inundation above\\nground level is possible in low lying areas near shorelines\\nand tidal waterways.\\n\\n* WHERE...Bayshore locations along San Francisco and Monterey\\nBay.\\n\\n* WHEN...For the Coastal Flood Advisory, until 3 PM PST Sunday.\\nFor the Beach Hazards Statement, through this evening.\\n\\n* IMPACTS...For the Beach Hazards Statement, sneaker waves can\\nunexpectedly run significantly farther up the beach than\\nnormal, including over rocks and jetties. Rip currents are\\ntypically more frequent and stronger in the vicinity of\\njetties, inlets, and piers. For the Coastal Flood Advisory,\\nflooding of lots, parks, and roads with only isolated road\\nclosures expected.\\n\\n* ADDITIONAL DETAILS...For the Coastal Flood Advisory, at the\\nSan Francisco tidal gauge high tide is expected to be 1.2 ft\\nabove normal (7.00 ft MLLW) at 9:04 AM Wednesday, 1.4 ft above\\nnormal (7.20 ft MLLW) at 9:48 AM Thursday, 1.4 ft above normal\\n(7.23 ft MLLW) at 10:35 AM Friday, 1.2 ft above normal (7.08\\nft MLLW) at 11:25 AM Saturday, and 0.9 ft above normal (6.75\\nft MLLW) at 12:17 PM Sunday. High tide timing varies up to 90\\nminutes earlier or later along the Pacific Coast and\\nthroughout the San Francisco Bay respectively.\",\n                \"instruction\": \"If travel is required, allow extra time as some roads may be\\nclosed. Do not drive around barricades or through water of\\nunknown depth. Take the necessary actions to protect flood-prone\\nproperty.\\n\\nDangerous conditions are forecast along the shoreline. Hazards\\ninclude sneaker waves, strong rip currents, and large breaking\\nwaves. Stay off the rocks and NEVER turn your back on the ocean!\",\n                \"response\": \"Avoid\",\n                \"parameters\": {\n                    \"AWIPSidentifier\": [\n                        \"CFWMTR\"\n                    ],\n                    \"WMOidentifier\": [\n                        \"WHUS46 KMTR 031153\"\n                    ],\n                    \"NWSheadline\": [\n                        \"COASTAL FLOOD ADVISORY REMAINS IN EFFECT UNTIL 3 PM PST SUNDAY... ...BEACH HAZARDS STATEMENT REMAINS IN EFFECT THROUGH THIS EVENING\"\n                    ],\n                    \"BLOCKCHANNEL\": [\n                        \"EAS\",\n                        \"NWEM\",\n                        \"CMAS\"\n                    ],\n                    \"VTEC\": [\n                        \"/O.CON.KMTR.BH.S.0021.000000T0000Z-251204T0600Z/\"\n                    ],\n                    \"eventEndingTime\": [\n                        \"2025-12-03T22:00:00-08:00\"\n                    ],\n                    \"expiredReferences\": [\n                        \"w-nws.webmaster@noaa.gov,urn:oid:2.49.0.1.840.0.08848c991336157878d38d1ffbfc9e9742984e52.001.2,2025-12-02T08:58:00-08:00 w-nws.webmaster@noaa.gov,urn:oid:2.49.0.1.840.0.af0dcb2190bc14836408315e4cc580c3d2cdeb53.001.2,2025-12-01T18:47:00-08:00 w-nws.webmaster@noaa.gov,urn:oid:2.49.0.1.840.0.21b1376d647bf4746e0a218223471eee19671728.001.1,2025-11-30T22:05:00-08:00 w-nws.webmaster@noaa.gov,urn:oid:2.49.0.1.840.0.1f8316f92149688b39489970d53bd68f7773609a.001.2,2025-11-30T18:54:00-08:00 w-nws.webmaster@noaa.gov,urn:oid:2.49.0.1.840.0.3f4b8992562fc7022a337464b529fc708f287fc3.001.1,2025-11-30T12:17:00-08:00 w-nws.webmaster@noaa.gov,urn:oid:2.49.0.1.840.0.ecd266091eb018733cf4fc9357c5c7fdae77a9b8.001.1,2025-11-30T01:28:00-08:00 w-nws.webmaster@noaa.gov,urn:oid:2.49.0.1.840.0.d12480d3eb90f5fecba0978dd9c1868b1693a420.001.1,2025-11-29T20:46:00-08:00 w-nws.webmaster@noaa.gov,urn:oid:2.49.0.1.840.0.a53d4d7f69e88a6370a59e3493ef574447077913.001.1,2025-11-29T07:30:00-08:00 w-nws.webmaster@noaa.gov,urn:oid:2.49.0.1.840.0.358cf61ddbf1745e21a67e3bba15ca0e524c2b41.001.1,2025-11-28T18:32:00-08:00 w-nws.webmaster@noaa.gov,urn:oid:2.49.0.1.840.0.7e8f6f91e5213f433eda0bb03a347f0857da0a39.001.1,2025-11-28T03:24:00-08:00\"\n                    ]\n                },\n                \"scope\": \"Public\",\n                \"code\": \"IPAWSv1.0\",\n                \"language\": \"en-US\",\n                \"web\": \"http://www.weather.gov\",\n                \"eventCode\": {\n                    \"SAME\": [\n                        \"NWS\"\n                    ],\n                    \"NationalWeatherService\": [\n                        \"BHS\"\n   
